vi "GVmotor_write_Pot_V0.vi"(8 "file_name":string="Pot_V0.txt", 11 "V0":dbl) -> ()   [LabVIEW 2019]
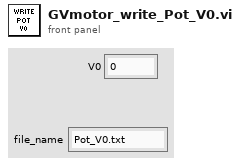
[diagram p1: front panel]
types:
  T1 = enum16{"open", "replace", "create", "open or create", "replace or create", "replace or create with confirmation"}
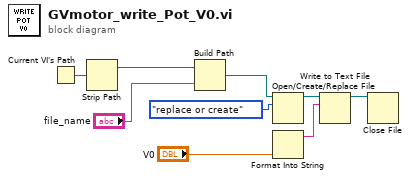
[diagram p0: block diagram]
diagram:
  n1 = Current VI's Path() -> (path=w5:path)
  n2 = Strip Path(path=w5) -> (stripped path=w4:path)  [unwired: 1 out]
  n3 = Build Path(base path=w4, name or relative path="file_name") -> (appended path=w3:path)
  n4 = Open/Create/Replace File(file path (use dialog)=w3, operation (0:open)=T1."replace or create") -> (refnum out=w8:refnum<file>)  [unwired: 4 in, 2 out]
  n5 = Format Into String("V0") -> (resulting string=w6:string)  [unwired: 3 in, 1 out]
  n6 = Write to Text File(file (use dialog)=w8, text=w6) -> (refnum out=w9:refnum<file>)  [unwired: 2 in, 2 out]
  n7 = Close File(refnum=w9) -> ()  [unwired: 1 in, 2 out]
